vi "GlobalVariable.vi"() -> ()   [LabVIEW 2020]
panel:
  in  "connection ID":refnum<k5>
  out "连机状态":bool
  out "V输出mbHR地址":u16[](array[numeric])
  out "电压输出":sgl[](array[numeric])
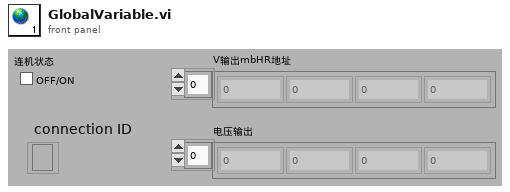
[diagram p1: front panel]
diagram:
